vi "imp_test_v7_9215.vi"() -> ()   [LabVIEW 2014]
uses:
  <vilib>/eio/EIONode/EIONode.xnode
  <vilib>/rvi/eio/common/nirviEmuTemplateMethod_errors.vi
  <vilib>/rvi/Analysis/measure/butterworth/XNode/niFpgaButterworthFilter.xnode
  <vilib>/rvi/DataTransferAndStorage/Container/XNode/niFpgaContainer.xnode
  <vilib>/rvi/FXPMathLib/FxpMul/XNode/nifxpmath_Multiplier.xnode
  <vilib>/rvi/FXPMathLib/sim/FxpSim.dll
  <vilib>/rvi/FXPMathLib/FxpSinAndCos/XNode/nifxpmath_SinAndCos.xnode
  <vilib>/rvi/FXPMathLib/FxpSinAndCos/simVIs/DllFxpSinAndCosTemp_sub.vi
  <vilib>/rvi/FXPMathLib/FxpSinAndCos/subVIs/nifxpmath_SinAndCos_SimConfig.ctl
  <vilib>/rvi/FXPMathLib/FxpSub/XNode/nifxpmath_Sub.xnode
  <vilib>/rvi/FXPMathLib/FxpAdd/XNode/nifxpmath_Add.xnode
  <vilib>/rvi/interface/RandomDataEmulation/nirviRandomDataFpgaMultiElementTemplate.vi
panel:
  out "Strain_y (Avg2 w. f)":fxp<+/-,34,7>
  in  "Strain_y Avg2 coeff.":i32[](array[numeric])=[946630756, 63555534]
  out "Strain_y (Avg4 w. f)":fxp<+/-,35,7>
  in  "Strain_y Avg4 coeff.":i32[](array[numeric])=[946630756, 63555534]
  out "Strain_y (Avg2)":fxp<+/-,30,3>
  out "Strain_y (Avg4)":fxp<+/-,31,3>
  in  "Belt_op":fxp<+/-,7,7>
  in  "Belt_mp":fxp<+/-,6,6>
  in  "Belt_oy":fxp<+/-,7,7>
  in  "Belt_my":fxp<+/-,6,6>
  out "Fp_dc":fxp<+/-,32,10>
  out "Fy_dc":fxp<+/-,32,10>
  in  "Zero_y":bool
  in  "Zero_p":bool
  in  "mt0_omega_p":u32
  in  "Encoder reset":bool
  out "fpt_d":fxp<+/-,36,18>
  out "Dp_error_dd":fxp<+/-,36,16>
  out "Dp_error_d":fxp<+/-,33,8>
  in  "Dp_dd coeff.":i32[](array[numeric])=[946630756, 63555534]
  out "Dp_dd":fxp<+/-,36,25>
  out "dFp_PID":fxp<+/-,36,18>
  in  "dFp_PID coeff.":i32[](array[numeric])=[946630756, 63555534]
  out "fpt_i":fxp<+/-,34,18>
  in  "Bv_p":fxp<+/-,22,8>
  in  "Kv_p":fxp<+/-,22,8>
  out "Dp_error":fxp<+/-,22,7>
  out "Dpr_sin":fxp<+/-,22,7>
  in  "Sin offset_p":fxp<+/-,22,7>
  in  "Sin magnitude_p":fxp<+/-,21,6>
  out "Dpr_sin_dd":fxp<+/-,35,20>
  out "Dpr_sin_d":fxp<+/-,33,15>
  out "Sin omega_p":fxp<+/-,34,9>
  in  "Sin wave freq._p (Hz)":fxp<+/-,32,6>
  in  "Dpr_step":fxp<+/-,22,7>
  out "Dpr_for":fxp<+/-,22,7>
  in  "Command_p":i16(ring) items=["Step", "Sine"]
  in  "Ki_p":fxp<+/-,36,9>
  out "Fp_PID":fxp<+/-,36,16>
  in  "fp_tolorance":fxp<+,22,6>
  out "fp_tilde":fxp<+/-,33,10>
  in  "Kd_p":fxp<+/-,36,9>
  in  "Kp_p":fxp<+/-,36,9>
  out "Fr_p":fxp<+/-,32,10>
  in  "S/F coeff_p":fxp<+/-,25,-10>
  in  "S/F coeff_y":fxp<+/-,25,-10>
  out "va_p":fxp<+/-,36,7>
  out "vb_p":fxp<+/-,37,8>
  out "vq_p_F":fxp<+/-,20,5> format="%.57g"
  out "vd_p_F":fxp<+/-,20,5>
  in  "dFp_add":bool
  in  "Stop motor_p":bool
  out "Force_p":fxp<+/-,32,10>
  in  "Strain selection_p":i16(ring) items=["Raw", "Avg.", "Avg. w. filter"]
  out "Strain_p (Avg w. f)":fxp<+/-,36,8>
  in  "Strain_p mean coeff.":i32[](array[numeric])=[946630756, 63555534]
  out "Strain_p (Avg)":fxp<+/-,36,4>
  out "Raw Strain_p":fxp<+/-,36,4>
  out "Mod6/AI3":fxp<+/-,36,4>
  in  "Strain gage reset_p":bool
  out "Dp_d (mm/s)":fxp<+/-,36,11>
  out "omega_p (rad/s)":fxp<+/-,20,9>
  out "mt_omega_p":u32
  out "rad_p(NrTheta)":fxp<+/-,33,20>
  out "D_p(mm)":fxp<+/-,32,7>
  out "Encoder Position_p":i32
  in  "Encoder reset_p":bool
  out "Strain_y (Avg8 w. f)":fxp<+/-,36,8>
  in  "Strain_y Avg8 coeff.":i32[](array[numeric])=[-898916953, 1957103773, 3888751]
  out "Dyr_for":fxp<+/-,22,7>
  in  "Command_y":i16(ring) items=["Step", "Sine"]
  out "Strain_y (Avg8)":fxp<+/-,36,4>
  in  "Strain selection_y":i16(ring) items=["Raw", "Avg.", "Avg. w. filter"]
  out "vb_y":fxp<+/-,38,8>
  out "va_y":fxp<+/-,38,8>
  out "fyt_d":fxp<+/-,36,18>
  out "Fr_y":fxp<+/-,32,10>
  in  "Bv_y":fxp<+/-,22,8>
  out "Dy_error_dd":fxp<+/-,36,16>
  out "Dy_error_d":fxp<+/-,33,8>
  in  "Kv_y":fxp<+/-,22,8>
  out "Dy_error":fxp<+/-,22,7>
  out "Dyr_sin_dd":fxp<+/-,35,20>
  out "Dyr_sin_d":fxp<+/-,33,15>
  out "Sin omega_y":fxp<+/-,34,9>
  out "Dyr_sin":fxp<+/-,22,7>
  in  "Sin offset_y":fxp<+/-,22,7>
  in  "Sin magnitude_y":fxp<+/-,21,6>
  out "Time now(s)":fxp<+,52,14>
  in  "Sin wave freq._y (Hz)":fxp<+/-,32,6>
  in  "Dyr_step":fxp<+/-,22,7>
  in  "Drive mode":i16(ring) items=["Backward", "Forward"]
  out "Dy_dd":fxp<+/-,36,25>
  in  "Dy_dd coeff.":i32[](array[numeric])=[946630756, 63555534]
  out "dFy_PID":fxp<+/-,36,18>
  in  "dFy_PID coeff.":i32[](array[numeric])=[946630756, 63555534]
  out "fyt_i":fxp<+/-,36,16>
  out "Fy_PID":fxp<+/-,36,16>
  in  "fy_tolorance":fxp<+,22,6>
  in  "Ki_y":fxp<+/-,36,9>
  in  "Kd_y":fxp<+/-,36,9>
  out "fy_tilde":fxp<+/-,32,10>
  in  "Kp_y":fxp<+/-,36,9>
  out "vq_y_F":fxp<+/-,20,5> format="%.57g"
  out "vd_y_F":fxp<+/-,20,5>
  in  "dFy_add":bool
  in  "Stop motor_y":bool
  out "Dy_d (mm/s)":fxp<+/-,36,11>
  out "omega_y (rad/s)":fxp<+/-,20,9>
  in  "mt0_omega_y":u32
  out "mt_omega_y":u32
  out "rad_y(NrTheta)":fxp<+/-,33,20>
  out "D_y(mm)":fxp<+/-,32,7>
  out "Encoder Position_y":i32
  in  "Encoder reset_y":bool
  in  "Ini coe.":bool
  out "Loop rate (kHz)":fxp<+/-,36,7>
  out "Force_y":fxp<+/-,32,10>
  out "Raw Strain_y":fxp<+/-,36,4>
  in  "Strain gage reset_y":bool
  out "Mod6/AI2":fxp<+/-,36,4>
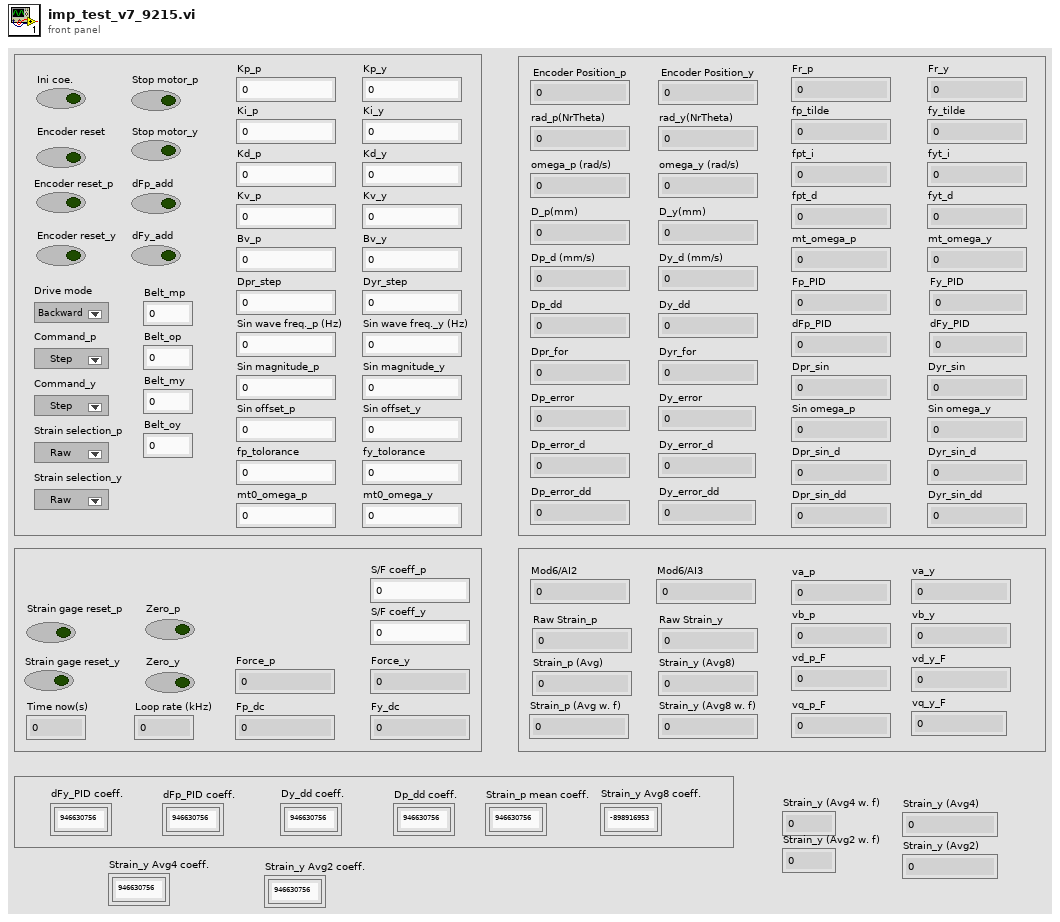
[diagram p1: front panel]
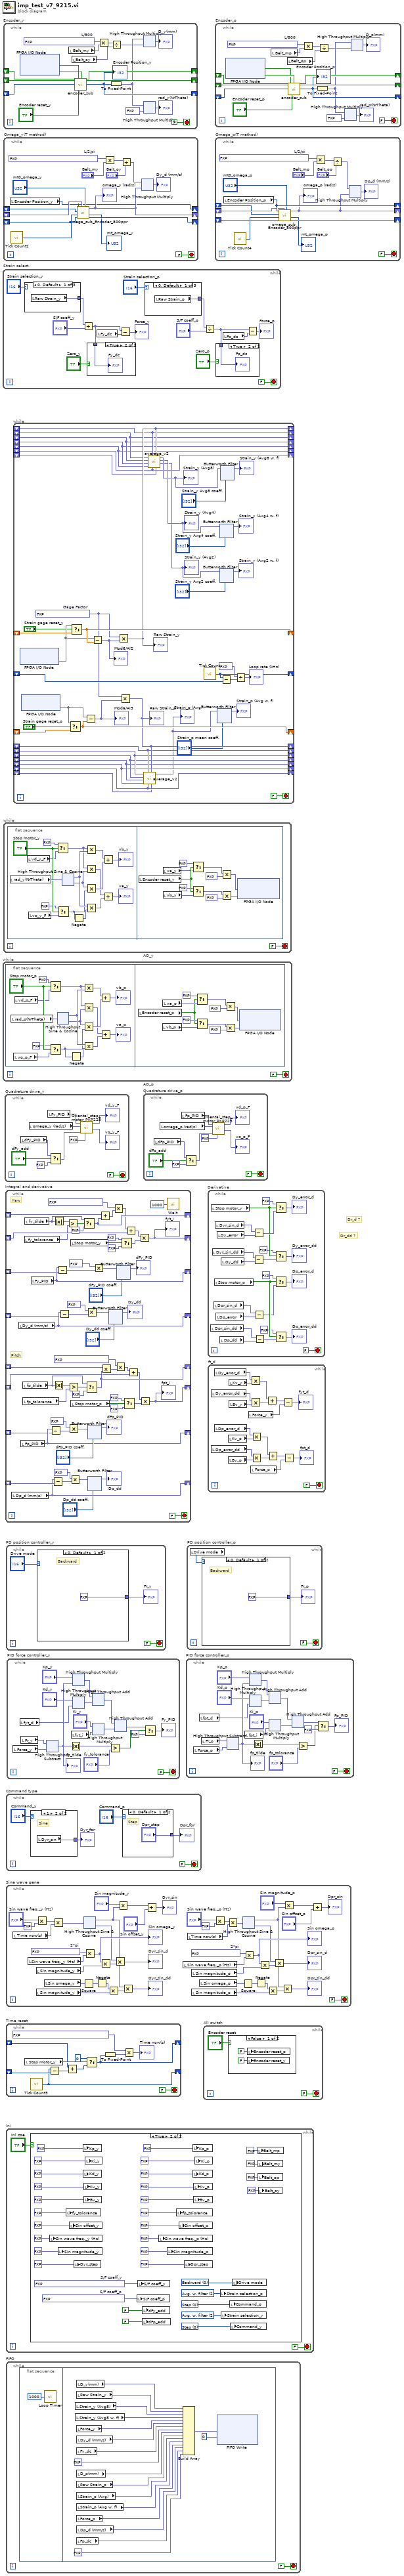
[diagram p0: block diagram]
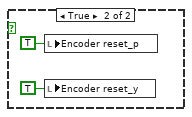
[diagram p2: hidden frame]
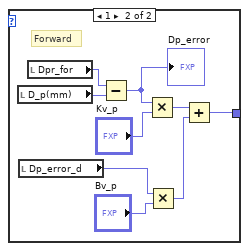
[diagram p3: hidden frame]
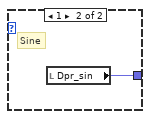
[diagram p4: hidden frame]
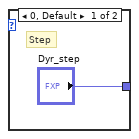
[diagram p5: hidden frame]
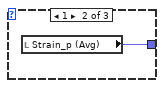
[diagram p8: hidden frame]
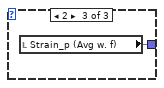
[diagram p9: hidden frame]
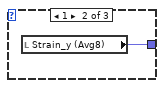
[diagram p10: hidden frame]
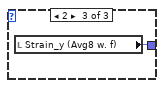
[diagram p11: hidden frame]
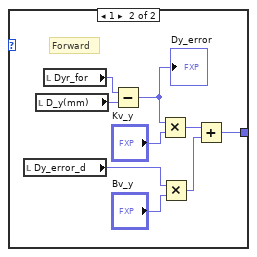
[diagram p12: hidden frame]
diagram:
  # "Dr_dd ?"
  # "Dr_d ?"
  n1 = while "Strain select." {
    stop <- FALSE stop-if-true
    n2 = case shown="0, Default" "Strain selection_y" {
      tunnel: [w21 w22 w23] -> w14
      frame 0, Default {
        n3 = local read "Raw Strain_y"() -> (w21:fxp<+/-,36,4>)
      }
      frame 1 {
        n4 = local read "Strain_y (Avg8)"() -> (w22:fxp<+/-,36,4>)
      }
      frame 2 {
        n5 = local read "Strain_y (Avg8 w. f)"() -> (w23:fxp<+/-,36,8>)
      }
    }
    n6 = Divide(x=w14, y="S/F coeff_y") -> (x/y=w7:fxp<+/-,32,10>)
    n7 = case shown="True" "Zero_y" {
      tunnel: w7 -> [_ w17]
      frame False {
      }
      frame True {
        "Fy_dc" <- w17
      }
    }
    n8 = local read "Fy_dc"() -> (w8:fxp<+/-,32,10>)
    n9 = Subtract(x=w7, y=w8) -> (x-y=→"Force_y":fxp<+/-,33,11>)
    n10 = case shown="0, Default" "Strain selection_p" {
      tunnel: [w18 w19 w20] -> w12
      frame 0, Default {
        n11 = local read "Raw Strain_p"() -> (w18:fxp<+/-,36,4>)
      }
      frame 1 {
        n12 = local read "Strain_p (Avg)"() -> (w19:fxp<+/-,36,4>)
      }
      frame 2 {
        n13 = local read "Strain_p (Avg w. f)"() -> (w20:fxp<+/-,36,8>)
      }
    }
    n14 = Divide(x=w12, y="S/F coeff_p") -> (x/y=w4:fxp<+/-,32,10>)
    n15 = case shown="True" "Zero_p" {
      tunnel: w4 -> [_ w16]
      frame False {
      }
      frame True {
        "Fp_dc" <- w16
      }
    }
    n16 = local read "Fp_dc"() -> (w2:fxp<+/-,32,10>)
    n17 = Subtract(x=w4, y=w2) -> (x-y=→"Force_p":fxp<+/-,33,11>)
  }
  n18 = while "AO_p" {
    stop <- FALSE stop-if-true
    n19 = flat-sequence {
      frame #0 {
        n20 = local read "rad_p(NrTheta)"() -> (w36:fxp<+/-,33,20>)
        n21 = local read "vq_p_F"() -> (w37:fxp<+/-,20,5>)
        n22 = local read "vd_p_F"() -> (w39:fxp<+/-,20,5>)
        n23 = Select(t=fxp<+/-,20,5> 0.0, s="Stop motor_p", f=w39) -> (s? t:f=w28:fxp<+/-,20,5>)
        n24 = Select(t=fxp<+,1,1> 0.0, s="Stop motor_p", f=w37) -> (s? t:f=w27:fxp<+/-,20,5>)
        n25 = xnode "High Throughput Sine & Cosine"("x (pi)"=w36) -> ("sin(x)"=w30:fxp<+/-,16,2>, "cos(x)"=w29:fxp<+/-,16,2>)
        n26 = Negate(x=w27) -> (-x=w35:fxp<+/-,21,6>)
        n27 = Multiply(x=w28, y=w30) -> (x*y=w34:fxp<+/-,36,7>)
        n28 = Multiply(x=w28, y=w29) -> (x*y=w32:fxp<+/-,36,7>)
        n29 = Multiply(x=w29, y=w27) -> (x*y=w33:fxp<+/-,36,7>)
        n30 = Multiply(x=w30, y=w35) -> (x*y=w31:fxp<+/-,35,6>)
        n31 = Add(x=w34, y=w33) -> (x+y=→"vb_p":fxp<+/-,37,8>)
        n32 = Add(x=w32, y=w31) -> (x+y=→"va_p":fxp<+/-,36,7>)
      }
      frame #1 {
        n33 = local read "Encoder reset_p"() -> (w72:bool)
        n34 = local read "vb_p"() -> (w73:fxp<+/-,37,8>)
        n35 = local read "va_p"() -> (w74:fxp<+/-,36,7>)
        n36 = Select(t=fxp<+,2,2> 3.0, s=w72, f=w74) -> (s? t:f=w80:fxp<+/-,36,7>)
        n37 = Select(t=fxp<+,1,1> 0.0, s=w72, f=w73) -> (s? t:f=w79:fxp<+/-,37,8>)
        n38 = Multiply(x=w80, y=fxp<+/-,1,0> -0.5) -> (x*y=w75:fxp<+/-,36,6>)
        n39 = Multiply(x=w79, y=fxp<+/-,1,0> -0.5) -> (x*y=w76:fxp<+/-,36,6>)
        n40 = xnode "FPGA I/O Node"("Mod8/AO0"=w75, "Mod8/AO1"=w76) -> ()  [unwired: 2 in, 2 out]
      }
    }
  }
  n41 = while "Encoder_y" {
    shift-right: [w98] -> _
    shift-left: _ -> [w99]
    shift-right: [w100] -> _
    shift-left: _ -> [w101]
    shift-right: [w93] -> _
    shift-left: _ -> [w97]
    stop <- FALSE stop-if-true
    w87 = fxp<+/-,20,-5> 0.002499997615814209  # L/800
    n42 = xnode "FPGA I/O Node"() -> ("Mod4/DI3"=w96:bool, "Mod4/DI4"=w95:bool)  [unwired: 2 in, 2 out]
    n43 = local read "Belt_my"() -> (w86:fxp<+/-,6,6>)
    n44 = local read "Belt_oy"() -> (w84:fxp<+/-,7,7>)
    n45 = call "encoder_sub.vi"("A_pre"=w99, "B_pre"=w101, "Encoder Position_pre"=w97, "A input"=w96, "Encoder Position Reset"="Encoder reset_y", "B input"=w95) -> ("A"=w98:bool, "B"=w100:bool, "Encoder Position (Counts)"=w93:i32)  [unwired: 19 in]
    "Encoder Position_y" <- w93
    n46 = Multiply(x=w87, y=w86) -> (x*y=w85:fxp<+/-,26,1>)
    n47 = To Fixed-Point(number=w93) -> (fixed-point=w92:fxp<+/-,32,32>)  [unwired: 1 in]
    n48 = Divide(x=w85, y=w84) -> (x/y=w83:fxp<+/-,33,1>)
    n49 = xnode ("High Throughput Multiply")("x"=w92, "y"=w83) -> ("x*y"=→"D_y(mm)":fxp<+/-,64,33>)
    n50 = xnode ("High Throughput Multiply")("x"=w92, "y"=fxp<+/-,16,1> 0.125) -> ("x*y"=→"rad_y(NrTheta)":fxp<+/-,48,33>)
  }
  n51 = while "AO_y" {
    stop <- FALSE stop-if-true
    n52 = flat-sequence {
      frame #0 {
        n53 = local read "rad_y(NrTheta)"() -> (w119:fxp<+/-,33,20>)
        n54 = local read "vd_y_F"() -> (w117:fxp<+/-,20,5>)
        n55 = local read "vq_y_F"() -> (w116:fxp<+/-,20,5>)
        n56 = Select(t=fxp<+/-,20,5> 0.0, s="Stop motor_y", f=w117) -> (s? t:f=w111:fxp<+/-,20,5>)
        n57 = Select(t=fxp<+/-,20,5> 0.0, s="Stop motor_y", f=w116) -> (s? t:f=w110:fxp<+/-,20,5>)
        n58 = xnode "High Throughput Sine & Cosine"("x (pi)"=w119) -> ("sin(x)"=w113:fxp<+/-,17,2>, "cos(x)"=w112:fxp<+/-,17,2>)
        n59 = Negate(x=w110) -> (-x=w109:fxp<+/-,21,6>)
        n60 = Multiply(x=w111, y=w113) -> (x*y=w108:fxp<+/-,37,7>)
        n61 = Multiply(x=w111, y=w112) -> (x*y=w106:fxp<+/-,37,7>)
        n62 = Multiply(x=w112, y=w110) -> (x*y=w107:fxp<+/-,37,7>)
        n63 = Multiply(x=w113, y=w109) -> (x*y=w105:fxp<+/-,36,6>)
        n64 = Add(x=w108, y=w107) -> (x+y=→"vb_y":fxp<+/-,38,8>)
        n65 = Add(x=w106, y=w105) -> (x+y=→"va_y":fxp<+/-,37,7>)
      }
      frame #1 {
        n66 = local read "Encoder reset_y"() -> (w152:bool)
        n67 = local read "va_y"() -> (w151:fxp<+/-,38,8>)
        n68 = local read "vb_y"() -> (w150:fxp<+/-,38,8>)
        n69 = Select(t=fxp<+,2,2> 3.0, s=w152, f=w151) -> (s? t:f=w156:fxp<+/-,38,8>)
        n70 = Select(t=fxp<+,1,1> 0.0, s=w152, f=w150) -> (s? t:f=w155:fxp<+/-,38,8>)
        n71 = Multiply(x=w156, y=fxp<+/-,1,0> -0.5) -> (x*y=w159:fxp<+/-,39,8>)
        n72 = Multiply(x=w155, y=fxp<+/-,1,0> -0.5) -> (x*y=w160:fxp<+/-,37,6>)
        n73 = xnode "FPGA I/O Node"("Mod8/AO2"=w159, "Mod8/AO3"=w160) -> ()  [unwired: 2 in, 2 out]
      }
    }
  }
  n74 = while "Omega_y(T method)" {
    shift-right: [w167] -> _
    shift-left: _ -> [w168]
    shift-right: [w170] -> _
    shift-left: _ -> [w172]
    shift-right: [w174] -> _
    shift-left: _ -> [w175]
    stop <- FALSE stop-if-true
    w165 = fxp<+/-,32,0> 0.3183098859153688  # L/2/pi
    n75 = local read "Encoder Position_y"() -> (w167:i32)
    n76 = call "Tick Count2"() -> ("Tick Count(Ticks)"=w176:u32)
    n77 = call "omega_sub_Encoder_800ppr.vi"("mt0"="mt0_omega_y", "omega_pre"=w172, "ticks_m_pre"=w175, "ticks"=w176, "count_pre"=w168, "count"=w167) -> ("ticks_m"=w174:u32, "mt"=→"mt_omega_y":u32, "omega"=w170:fxp<+/-,20,9>)  [unwired: 3 in]
    "omega_y (rad/s)" <- w170
    n78 = Multiply(x=w165, y="Belt_my") -> (x*y=w163:fxp<+/-,38,6>)
    n79 = Divide(x=w163, y="Belt_oy") -> (x/y=w161:fxp<+/-,20,1>)
    n80 = xnode ("High Throughput Multiply")("x"=w161, "y"=w170) -> ("x*y"=→"Dy_d (mm/s)":fxp<+/-,40,10>)
  }
  n81 = while "Quadrature drive_y" {
    stop <- FALSE stop-if-true
    n82 = local read "dFy_PID"() -> (w178:fxp<+/-,36,18>)
    n83 = local read "omega_y (rad/s)"() -> (w186:fxp<+/-,20,9>)
    n84 = local read "Fy_PID"() -> (w179:fxp<+/-,36,16>)
    n85 = Select(t=w178, s="dFy_add", f=fxp<+,1,1> 0.0) -> (s? t:f=w182:fxp<+/-,36,18>)
    n86 = call "Oriental_step_motor_PKP225.vi"("F_Threshold"=fxp<+,12,12> 10.0, "dFmr"=w182, "omega"=w186, "Fmr"=w179) -> ("vq_F"=→"vq_y_F":fxp<+/-,20,5>, "vd_F"=→"vd_y_F":fxp<+/-,20,5>)  [unwired: 6 in]
  }
  n87 = while "Integral and derivative" {
    shift-right: [w242] -> _
    shift-left: _ -> [w241]
    shift-right: [w234] -> _
    shift-left: _ -> [w233]
    shift-right: [w244] -> _
    shift-left: _ -> [w245]
    shift-right: [w224] -> _
    shift-left: _ -> [w223]
    shift-right: [w210] -> _
    shift-left: _ -> [w213]
    shift-right: [w203] -> _
    shift-left: _ -> [w202]
    shift-right: [w197] -> _
    shift-left: _ -> [w196]
    shift-right: [w192] -> _
    shift-left: _ -> [w193]
    stop <- FALSE stop-if-true
    # "Pitch"
    # "Yaw"
    n88 = local read "Dp_d (mm/s)"() -> (w192:fxp<+/-,36,11>)
    n89 = local read "Dy_d (mm/s)"() -> (w224:fxp<+/-,36,11>)
    n90 = local read "Fp_PID"() -> (w197:fxp<+/-,36,16>)
    n91 = local read "fp_tilde"() -> (w214:fxp<+/-,33,10>)
    n92 = local read "fp_tolorance"() -> (w217:fxp<+,22,6>)
    n93 = local read "fy_tolorance"() -> (w220:fxp<+,22,6>)
    n94 = local read "fy_tilde"() -> (w246:fxp<+/-,32,10>)
    n95 = local read "Fy_PID"() -> (w244:fxp<+/-,36,16>)
    n96 = Subtract(x=w197, y=w196) -> (x-y=w201:fxp<+/-,37,17>)
    n97 = Subtract(x=w192, y=w193) -> (x-y=w194:fxp<+/-,37,12>)
    n98 = Absolute Value(x=w214) -> (abs(x)=w218:fxp<+,33,10>)
    n99 = Absolute Value(x=w246) -> (abs(x)=w248:fxp<+,32,10>)
    n100 = Subtract(x=w244, y=w245) -> (x-y=w232:fxp<+/-,37,17>)
    n101 = Subtract(x=w224, y=w223) -> (x-y=w226:fxp<+/-,36,11>)
    n102 = Greater?(x=w248, y=w220) -> (0:w249:bool)
    n103 = Greater?(x=w218, y=w217) -> (0:w216:bool)
    n104 = Multiply(x=fxp<+,7,10> 1000.0, y=w201) -> (x*y=w199:fxp<+/-,32,18>)
    n105 = Multiply(x=fxp<+,7,10> 1000.0, y=w194) -> (x*y=w190:fxp<+/-,36,21>)
    n106 = local read "Stop motor_y"() -> (w235:bool)
    n107 = local read "Stop motor_p"() -> (w205:bool)
    n108 = Select(t=w246, s=w249, f=fxp<+/-,33,11> 0.0) -> (s? t:f=w242:fxp<+/-,33,11>)
    n109 = Select(t=w214, s=w216, f=fxp<+,1,1> 0.0) -> (s? t:f=w210:fxp<+/-,33,10>)
    n110 = Multiply(x=fxp<+,7,10> 1000.0, y=w226) -> (x*y=w225:fxp<+/-,36,21>)
    n111 = xnode "Butterworth Filter"("input data"=w199, "scaled coefficients"="dFp_PID coeff.") -> ("output data"=→"dFp_PID":fxp<+/-,36,22>)  [unwired: 1 in]
    n112 = xnode "Butterworth Filter"("input data"=w190, "scaled coefficients"="Dp_dd coeff.") -> ("output data"=→"Dp_dd":fxp<+/-,36,25>)  [unwired: 1 in]
    n113 = Multiply(x=fxp<+,7,10> 1000.0, y=w232) -> (x*y=w229:fxp<+/-,32,18>)
    n114 = Add(x=w241, y=w242) -> (x+y=w247:fxp<+/-,34,12>)
    n115 = Multiply(x=w213, y=w210) -> (x*y=w212:fxp<+/-,34,12>)
    n116 = xnode "Butterworth Filter"("input data"=w225, "scaled coefficients"="Dy_dd coeff.") -> ("output data"=→"Dy_dd":fxp<+/-,36,25>)  [unwired: 1 in]
    n117 = Multiply(x=fxp<+/-,30,12> 0.000499725341796875, y=w247) -> (x*y=w240:fxp<+/-,34,10>)
    n118 = Multiply(x=fxp<+/-,30,12> 0.000499725341796875, y=w212) -> (x*y=w209:fxp<+/-,34,10>)
    n119 = xnode "Butterworth Filter"("input data"=w229, "scaled coefficients"="dFy_PID coeff.") -> ("output data"=→"dFy_PID":fxp<+/-,36,22>)  [unwired: 1 in]
    n120 = Select(t=fxp<+,1,1> 0.0, s=w235, f=fxp<+,1,1> 1.0) -> (s? t:f=w238:fxp<+,1,1>)
    n121 = Select(t=fxp<+,1,1> 0.0, s=w205, f=fxp<+,1,1> 1.0) -> (s? t:f=w207:fxp<+,1,1>)
    n122 = Add(x=w240, y=w233) -> (x+y=w239:fxp<+/-,36,16>)
    n123 = Add(x=w209, y=w202) -> (x+y=w208:fxp<+/-,36,16>)
    n124 = Multiply(x=w239, y=w238) -> (x*y=w234:fxp<+/-,34,18>)
    "fyt_i" <- w234
    n125 = Multiply(x=w208, y=w207) -> (x*y=w203:fxp<+/-,34,18>)
    "fpt_i" <- w203
    n126 = call "Wait"("Count(uSec)"=u32 1000) -> ()  [unwired: 1 out]
  }
  n127 = while "PD position controller_y" {
    stop <- FALSE stop-if-true
    n128 = case shown="0, Default" "Drive mode" {
      tunnel: [fxp<+/-,62,19> 0.0 w288] -> w284
      frame 0, Default {
        # "Backward"
      }
      frame 1 {
        # "Forward"
        n129 = local read "Dy_error_d"() -> (w290:fxp<+/-,33,8>)
        n130 = local read "D_y(mm)"() -> (w295:fxp<+/-,32,7>)
        n131 = local read "Dyr_for"() -> (w287:fxp<+/-,22,7>)
        n132 = Subtract(x=w287, y=w295) -> (x-y=w294:fxp<+/-,33,8>)
        "Dy_error" <- w294
        n133 = Multiply(x=w294, y="Kv_y") -> (x*y=w292:fxp<+/-,54,15>)
        n134 = Multiply(x=w290, y="Bv_y") -> (x*y=w289:fxp<+/-,55,16>)
        n135 = Add(x=w292, y=w289) -> (x+y=w288:fxp<+/-,55,16>)
      }
    }
    "Fr_y" <- w284
  }
  n136 = while "Command type" {
    stop <- FALSE stop-if-true
    n137 = case shown="1" "Command_y" {
      tunnel: ["Dyr_step" w304] -> w299
      frame 0, Default {
        # "Step"
      }
      frame 1 {
        # "Sine"
        n138 = local read "Dyr_sin"() -> (w304:fxp<+/-,22,7>)
      }
    }
    "Dyr_for" <- w299
    n139 = case shown="0, Default" "Command_p" {
      tunnel: ["Dpr_step" w302] -> w297
      frame 0, Default {
        # "Step"
      }
      frame 1 {
        # "Sine"
        n140 = local read "Dpr_sin"() -> (w302:fxp<+/-,22,7>)
      }
    }
    "Dpr_for" <- w297
  }
  n141 = while "Sine wave gene" {
    stop <- FALSE stop-if-true
    w310 = fxp<+,20,3> 6.2831878662109375  # 2*pi
    w342 = fxp<+,20,3> 6.2831878662109375  # 2*pi
    n142 = local read "Time now(s)"() -> (w348:fxp<+,52,14>)
    n143 = local read "Sin wave freq._y (Hz)"() -> (w341:fxp<+/-,32,6>)
    n144 = Multiply(x="Sin wave freq._y (Hz)", y=fxp<+/-,10,3> 2.0) -> (x*y=w349:fxp<+/-,41,9>)
    n145 = local read "Sin magnitude_y"() -> (w339:fxp<+/-,21,6>)
    n146 = local read "Sin magnitude_y"() -> (w332:fxp<+/-,21,6>)
    n147 = local read "Sin omega_y"() -> (w335:fxp<+/-,34,9>)
    n148 = Multiply(x=w349, y=w348) -> (x*y=w347:fxp<+/-,41,19>)
    n149 = Square(x=w335) -> (x^2=w334:fxp<+,34,18>)
    n150 = xnode "High Throughput Sine & Cosine"("x (pi)"=w347) -> ("sin(x)"=w329:fxp<+/-,16,2>, "cos(x)"=w337:fxp<+/-,16,2>)
    n151 = Multiply(x=w342, y=w341) -> (x*y=w340:fxp<+/-,34,9>)
    "Sin omega_y" <- w340
    n152 = Negate(x=w334) -> (-x=w333:fxp<+/-,35,19>)
    n153 = Multiply(x=w340, y=w339) -> (x*y=w338:fxp<+/-,33,15>)
    n154 = Multiply(x=w333, y=w332) -> (x*y=w331:fxp<+/-,34,20>)
    n155 = Multiply(x=w337, y=w338) -> (x*y=→"Dyr_sin_d":fxp<+/-,33,15>)
    n156 = Multiply(x="Sin magnitude_y", y=w329) -> (x*y=w345:fxp<+/-,37,8>)
    n157 = Multiply(x=w329, y=w331) -> (x*y=→"Dyr_sin_dd":fxp<+/-,35,20>)
    n158 = Add(x=w345, y="Sin offset_y") -> (x+y=→"Dyr_sin":fxp<+/-,37,8>)
    n159 = local read "Sin wave freq._p (Hz)"() -> (w306:fxp<+/-,32,6>)
    n160 = local read "Time now(s)"() -> (w324:fxp<+,52,14>)
    n161 = local read "Sin magnitude_p"() -> (w307:fxp<+/-,21,6>)
    n162 = local read "Sin magnitude_p"() -> (w309:fxp<+/-,21,6>)
    n163 = local read "Sin omega_p"() -> (w308:fxp<+/-,34,9>)
    n164 = Multiply(x="Sin wave freq._p (Hz)", y=fxp<+/-,10,3> 2.0) -> (x*y=w328:fxp<+/-,42,9>)
    n165 = Multiply(x=w328, y=w324) -> (x*y=w325:fxp<+/-,41,19>)
    n166 = Square(x=w308) -> (x^2=w320:fxp<+,34,18>)
    n167 = xnode "High Throughput Sine & Cosine"("x (pi)"=w325) -> ("sin(x)"=w311:fxp<+/-,16,2>, "cos(x)"=w316:fxp<+/-,16,2>)
    n168 = Multiply(x=w310, y=w306) -> (x*y=w323:fxp<+/-,34,9>)
    "Sin omega_p" <- w323
    n169 = Negate(x=w320) -> (-x=w319:fxp<+/-,35,19>)
    n170 = Multiply(x=w323, y=w307) -> (x*y=w322:fxp<+/-,33,15>)
    n171 = Multiply(x=w319, y=w309) -> (x*y=w318:fxp<+/-,35,19>)
    n172 = Multiply(x=w316, y=w322) -> (x*y=→"Dpr_sin_d":fxp<+/-,33,15>)
    n173 = Multiply(x=w311, y=w318) -> (x*y=→"Dpr_sin_dd":fxp<+/-,35,20>)
    n174 = Multiply(x="Sin magnitude_p", y=w311) -> (x*y=w314:fxp<+/-,37,8>)
    n175 = Add(x=w314, y="Sin offset_p") -> (x+y=→"Dpr_sin":fxp<+/-,37,8>)
  }
  n176 = while "Time reset" {
    shift-right: [w421] -> _
    shift-left: _ -> [w422]
    shift-right: [w416] -> _
    shift-left: _ -> [w417]
    stop <- FALSE stop-if-true
    n177 = local read "Stop motor_y"() -> (w423:bool)
    n178 = call "Tick Count3"() -> ("Tick Count(uSec)"=w421:u32)
    n179 = Subtract(x=w421, y=w422) -> (x-y=w420:u32)
    n180 = Add(x=w417, y=w420) -> (x+y=w419:u32)
    n181 = Select(t=u32 0, s=w423, f=w419) -> (s? t:f=w416:u32)
    n182 = To Fixed-Point(number=w416) -> (fixed-point=w415:fxp<+,32,32>)  [unwired: 1 in]
    n183 = Multiply(x=fxp<+,20,-18> 1.0000003385357559e-06, y=w415) -> (x*y=→"Time now(s)":fxp<+,52,14>)
  }
  n184 = while "Ini" {
    stop <- FALSE stop-if-true
    n185 = case shown="True" "Ini coe." {
      frame False {
      }
      frame True {
        w441 = i16 0 items=["Step", "Sine"] ("Command_p")
        w442 = i16 2 items=["Raw", "Avg.", "Avg. w. filter"] ("Strain selection_p")
        w443 = i16 0 items=["Step", "Sine"] ("Command_y")
        w444 = i16 2 items=["Raw", "Avg.", "Avg. w. filter"] ("Strain selection_y")
        w446 = fxp<+/-,25,-10> -5.851034075021744e-07  # S/F coeff_p
        w445 = fxp<+/-,25,-10> -1.0477961041033268e-06  # S/F coeff_y
        w452 = i16 0 items=["Backward", "Forward"] ("Drive mode")
        n186 = local write "Sin wave freq._y (Hz)"(fxp<+/-,32,6> 1.0 ("Sin wave freq. (Hz)")) -> ()
        n187 = local write "Sin magnitude_y"(fxp<+/-,22,7> 5.0 ("Sin magnitude")) -> ()
        n188 = local write "fy_tolorance"(fxp<+,22,6> 5.0 ("f_tolorance")) -> ()
        n189 = local write "Sin offset_y"(fxp<+/-,38,9> 0.0 ("Sin offset")) -> ()
        n190 = local write "Dyr_step"(fxp<+/-,22,7> 0.0 ("Dr")) -> ()
        n191 = local write "Kp_y"(fxp<+/-,36,9> 30.0 ("Kp")) -> ()
        n192 = local write "Kd_y"(fxp<+/-,36,9> 0.0 ("Kd")) -> ()
        n193 = local write "Kv_y"(fxp<+/-,22,8> 0.0 ("Kv")) -> ()
        n194 = local write "Bv_y"(fxp<+/-,22,8> 0.0 ("Bv")) -> ()
        n195 = local write "Ki_y"(fxp<+/-,36,9> 0.0 ("Ki")) -> ()
        n196 = local write "S/F coeff_p"(w446) -> ()
        n197 = local write "S/F coeff_y"(w445) -> ()
        n198 = local write "dFy_add"(FALSE ("dF_add")) -> ()
        n199 = local write "dFp_add"(FALSE ("dFp_add")) -> ()
        n200 = local write "Sin wave freq._p (Hz)"(fxp<+/-,32,6> 1.0 ("Sin wave freq._p (Hz)")) -> ()
        n201 = local write "Sin magnitude_p"(fxp<+/-,21,6> 5.0 ("Sin magnitude_p")) -> ()
        n202 = local write "fp_tolorance"(fxp<+,22,6> 5.0 ("fp_tolorance")) -> ()
        n203 = local write "Sin offset_p"(fxp<+/-,22,7> 0.0 ("Sin offset_p")) -> ()
        n204 = local write "Dpr_step"(fxp<+/-,22,7> 0.0 ("Dpr_step")) -> ()
        n205 = local write "Kp_p"(fxp<+/-,36,9> 30.0 ("Kp_p")) -> ()
        n206 = local write "Kd_p"(fxp<+/-,36,9> 0.0 ("Kd_p")) -> ()
        n207 = local write "Kv_p"(fxp<+/-,22,8> 0.0 ("Kv_p")) -> ()
        n208 = local write "Bv_p"(fxp<+/-,22,8> 0.0 ("Bv_p")) -> ()
        n209 = local write "Ki_p"(fxp<+/-,36,9> 0.0 ("Ki_p")) -> ()
        n210 = local write "Strain selection_p"(w442) -> ()
        n211 = local write "Strain selection_y"(w444) -> ()
        n212 = local write "Command_p"(w441) -> ()
        n213 = local write "Command_y"(w443) -> ()
        n214 = local write "Drive mode"(w452) -> ()
        n215 = local write "Belt_mp"(fxp<+/-,6,6> 16.0 ("Belt_mp")) -> ()
        n216 = local write "Belt_my"(fxp<+/-,6,6> 22.0 ("Belt_my")) -> ()
        n217 = local write "Belt_op"(fxp<+/-,7,7> 16.0 ("Belt_op")) -> ()
        n218 = local write "Belt_oy"(fxp<+/-,7,7> 22.0 ("Belt_oy")) -> ()
      }
    }
  }
  n219 = while "FIFO" {
    stop <- FALSE stop-if-true
    n220 = flat-sequence {
      frame #0 {
        n221 = call "Loop Timer"("Count(uSec)"=u32 1000) -> ()  [unwired: 1 out]
      }
      frame #1 {
        n222 = local read "Strain_y (Avg8)"() -> (w476:fxp<+/-,36,4>)
        n223 = local read "Strain_y (Avg8 w. f)"() -> (w475:fxp<+/-,36,8>)
        n224 = local read "D_y(mm)"() -> (w478:fxp<+/-,32,7>)
        n225 = local read "Raw Strain_y"() -> (w477:fxp<+/-,36,4>)
        n226 = local read "Force_y"() -> (w470:fxp<+/-,32,10>)
        n227 = local read "Dy_d (mm/s)"() -> (w471:fxp<+/-,36,11>)
        n228 = local read "Fy_dc"() -> (w472:fxp<+/-,32,10>)
        n229 = local read "D_p(mm)"() -> (w469:fxp<+/-,32,7>)
        n230 = local read "Raw Strain_p"() -> (w468:fxp<+/-,36,4>)
        n231 = local read "Strain_p (Avg)"() -> (w467:fxp<+/-,36,4>)
        n232 = local read "Strain_p (Avg w. f)"() -> (w466:fxp<+/-,36,8>)
        n233 = local read "Force_p"() -> (w465:fxp<+/-,32,10>)
        n234 = local read "Dp_d (mm/s)"() -> (w464:fxp<+/-,36,11>)
        n235 = local read "Fp_dc"() -> (w463:fxp<+/-,32,10>)
        n236 = Build Array(w478, w477, w476, w475, w470, w471, w472, fxp<+/-,40,8> 0.0 ("element"), w469, w468, w467, w466, w465, w464, w463, fxp<+/-,40,8> 0.0 ("element")) -> (w461:fxp<+/-,43,11>[])
        n237 = xnode ("FIFO Write")("Element"=w461, "Timeout"=0) -> ()  [unwired: 1 in, 2 out]
      }
    }
  }
  n238 = while "PID force controller_y" {
    stop <- FALSE stop-if-true
    n239 = local read "Force_y"() -> (w496:fxp<+/-,32,10>)
    n240 = local read "fyt_d"() -> (w480:fxp<+/-,36,18>)
    n241 = local read "Fr_y"() -> (w482:fxp<+/-,32,10>)
    n242 = xnode "High Throughput Subtract"("x"=w482, "y"=w496) -> ("x-y"=w495:fxp<+/-,33,11>)
    "fy_tilde" <- w495
    n243 = Absolute Value(x=w495) -> (abs(x)=w486:fxp<+,33,11>)
    n244 = local read "fyt_i"() -> (w481:fxp<+/-,36,16>)
    n245 = xnode ("High Throughput Multiply")("x"="Kp_y", "y"=w495) -> ("x*y"=w493:fxp<+/-,64,20>)
    n246 = xnode ("High Throughput Multiply")("x"="Kd_y", "y"=w480) -> ("x*y"=w492:fxp<+/-,64,27>)
    n247 = xnode ("High Throughput Add")("x"=w493, "y"=w492) -> ("x+y"=w489:fxp<+/-,64,28>)
    n248 = xnode ("High Throughput Multiply")("x"="Ki_y", "y"=w481) -> ("x*y"=w490:fxp<+/-,64,25>)
    n249 = Greater?(x=w486, y="fy_tolorance") -> (0:w484:bool)
    n250 = xnode ("High Throughput Add")("x"=w489, "y"=w490) -> ("x+y"=w488:fxp<+/-,64,29>)
    n251 = Select(t=w488, s=w484, f=fxp<+/-,51,14> 0.0) -> (s? t:f=→"Fy_PID":fxp<+/-,64,29>)
  }
  n252 = while {
    shift-right: [w541] -> _
    shift-left: _ -> [w542]
    shift-right: [w537] -> _
    shift-left: _ -> [w538]
    shift-right: [w532] -> _
    shift-left: _ -> [w531]
    shift-right: [w531] -> _
    shift-left: _ -> [w530]
    shift-right: [w530] -> _
    shift-left: _ -> [w529]
    shift-right: [w529] -> _
    shift-left: _ -> [w528]
    shift-right: [w528] -> _
    shift-left: _ -> [w527]
    shift-right: [w527] -> _
    shift-left: _ -> [w526]
    shift-right: [w526] -> _
    shift-left: _ -> [w525]
    shift-right: [w519] -> _
    shift-left: _ -> [w520]
    shift-right: [w515] -> _
    shift-left: _ -> [w514]
    shift-right: [w514] -> _
    shift-left: _ -> [w513]
    shift-right: [w513] -> _
    shift-left: _ -> [w512]
    shift-right: [w512] -> _
    shift-left: _ -> [w511]
    shift-right: [w511] -> _
    shift-left: _ -> [w510]
    shift-right: [w510] -> _
    shift-left: _ -> [w509]
    shift-right: [w509] -> _
    shift-left: _ -> [w508]
    stop <- FALSE stop-if-true
    w517 = fxp<+,20,2> 2.115001678466797  # Gage Factor
    n253 = xnode "FPGA I/O Node"() -> ("Mod1/AI1"=w539)  [unwired: 2 in, 2 out]
    n254 = xnode "FPGA I/O Node"() -> ("Mod1/AI2"=w518)  [unwired: 2 in, 2 out]
    n255 = Select(t=w518, s="Strain gage reset_p", f=w520) -> (s? t:f=w519:dbl)
    n256 = Select(t=w539, s="Strain gage reset_y", f=w542) -> (s? t:f=w541:dbl)
    n257 = Subtract(x=w518, y=w519) -> (x-y=w516:fxp<+/-,30,-3>)
    "Mod6/AI3" <- w516
    n258 = Subtract(x=w539, y=w541) -> (x-y=w540:fxp<+/-,30,-3>)
    "Mod6/AI2" <- w540
    n259 = Multiply(x=w517, y=w540) -> (x*y=w532:fxp<+/-,41,6>)
    "Raw Strain_y" <- w532
    n260 = Multiply(x=w517, y=w516) -> (x*y=w515:fxp<+/-,50,-1>)
    "Raw Strain_p" <- w515
    n261 = call "average_v2.vi"("Numeric 8"=w508, "Numeric"=w515, "Numeric 7"=w509, "Numeric 2"=w514, "Numeric 6"=w510, "Numeric 5"=w511, "Numeric 4"=w512, "Numeric 3"=w513) -> ("Mean (8pt)"=w507:fxp<+/-,32,4>)  [unwired: 1 in, 2 out]
    "Strain_p (Avg)" <- w507
    n262 = call "average_v2.vi"("Numeric 8"=w525, "Numeric"=w532, "Numeric 7"=w526, "Numeric 2"=w531, "Numeric 6"=w527, "Numeric 5"=w528, "Numeric 4"=w529, "Numeric 3"=w530) -> ("Mean (2pt)"=w501:fxp<+/-,30,3>, "Mean (4pt)"=w504:fxp<+/-,31,3>, "Mean (8pt)"=w524:fxp<+/-,32,4>)  [unwired: 1 in]
    "Strain_y (Avg8)" <- w524
    "Strain_y (Avg4)" <- w504
    "Strain_y (Avg2)" <- w501
    n263 = call "Tick Count"() -> ("Tick Count(uSec)"=w537:u32)
    n264 = xnode "Butterworth Filter"("input data"=w507, "scaled coefficients"="Strain_p mean coeff.") -> ("output data"=→"Strain_p (Avg w. f)":fxp<+/-,36,8>)  [unwired: 1 in]
    n265 = xnode "Butterworth Filter"("input data"=w504, "scaled coefficients"="Strain_y Avg4 coeff.") -> ("output data"=→"Strain_y (Avg4 w. f)":fxp<+/-,35,7>)  [unwired: 1 in]
    n266 = xnode "Butterworth Filter"("input data"=w501, "scaled coefficients"="Strain_y Avg2 coeff.") -> ("output data"=→"Strain_y (Avg2 w. f)":fxp<+/-,34,7>)  [unwired: 1 in]
    n267 = xnode "Butterworth Filter"("input data"=w524, "scaled coefficients"="Strain_y Avg8 coeff.") -> ("output data"=→"Strain_y (Avg8 w. f)":fxp<+/-,32,4>)  [unwired: 1 in]
    n268 = Subtract(x=w537, y=w538) -> (x-y=w535:fxp<+/-,32,16>)
    n269 = Divide(x=fxp<+,7,10> 1000.0, y=w535) -> (x/y=→"Loop rate (kHz)":fxp<+/-,40,27>)
  }
  n270 = while "Quadrature drive_p" {
    stop <- FALSE stop-if-true
    n271 = local read "dFp_PID"() -> (w576:fxp<+/-,36,18>)
    n272 = local read "omega_p (rad/s)"() -> (w582:fxp<+/-,20,9>)
    n273 = local read "Fp_PID"() -> (w577:fxp<+/-,36,16>)
    n274 = Select(t=w576, s="dFp_add", f=fxp<+,1,1> 0.0) -> (s? t:f=w580:fxp<+/-,36,18>)
    n275 = call "Oriental_step_motor_PKP225.vi"("F_Threshold"=fxp<+,12,12> 10.0, "dFmr"=w580, "omega"=w582, "Fmr"=w577) -> ("vq_F"=→"vq_p_F":fxp<+/-,20,5>, "vd_F"=→"vd_p_F":fxp<+/-,20,5>)  [unwired: 6 in]
  }
  n276 = while "PID force controller_p" {
    stop <- FALSE stop-if-true
    n277 = local read "Force_p"() -> (w597:fxp<+/-,32,10>)
    n278 = local read "fpt_d"() -> (w588:fxp<+/-,36,18>)
    n279 = local read "Fr_p"() -> (w598:fxp<+/-,32,10>)
    n280 = xnode "High Throughput Subtract"("x"=w598, "y"=w597) -> ("x-y"=w589:fxp<+/-,33,11>)
    "fp_tilde" <- w589
    n281 = local read "fpt_i"() -> (w586:fxp<+/-,34,18>)
    n282 = xnode ("High Throughput Multiply")("x"="Kp_p", "y"=w589) -> ("x*y"=w587:fxp<+/-,64,20>)
    n283 = xnode ("High Throughput Multiply")("x"="Kd_p", "y"=w588) -> ("x*y"=w603:fxp<+/-,64,27>)
    n284 = Absolute Value(x=w589) -> (abs(x)=w596:fxp<+,33,11>)
    n285 = xnode ("High Throughput Add")("x"=w587, "y"=w603) -> ("x+y"=w601:fxp<+/-,64,28>)
    n286 = xnode ("High Throughput Multiply")("x"="Ki_p", "y"=w586) -> ("x*y"=w602:fxp<+/-,64,27>)
    n287 = xnode ("High Throughput Add")("x"=w601, "y"=w602) -> ("x+y"=w592:fxp<+/-,64,29>)
    n288 = Greater?(x=w596, y="fp_tolorance") -> (0:w593:bool)
    n289 = Select(t=w592, s=w593, f=fxp<+,1,1> 0.0) -> (s? t:f=→"Fp_PID":fxp<+/-,64,29>)
  }
  n290 = while "PD position controller_p" {
    stop <- FALSE stop-if-true
    n291 = local read "Drive mode"() -> (w606:i16)
    n292 = case shown="0, Default" w606 {
      tunnel: [fxp<+/-,62,19> 0.0 w609] -> w605
      frame 0, Default {
        # "Backward"
      }
      frame 1 {
        # "Forward"
        n293 = local read "D_p(mm)"() -> (w616:fxp<+/-,32,7>)
        n294 = local read "Dp_error_d"() -> (w608:fxp<+/-,33,8>)
        n295 = local read "Dpr_for"() -> (w615:fxp<+/-,22,7>)
        n296 = Subtract(x=w615, y=w616) -> (x-y=w614:fxp<+/-,24,8>)
        "Dp_error" <- w614
        n297 = Multiply(x=w614, y="Kv_p") -> (x*y=w611:fxp<+/-,34,16>)
        n298 = Multiply(x=w608, y="Bv_p") -> (x*y=w610:fxp<+/-,55,16>)
        n299 = Add(x=w611, y=w610) -> (x+y=w609:fxp<+/-,56,17>)
      }
    }
    "Fr_p" <- w605
  }
  n300 = while "All switch" {
    stop <- FALSE stop-if-true
    n301 = case shown="False" "Encoder reset" {
      frame False {
        n302 = local write "Encoder reset_p"(FALSE ("Encoder reset_p")) -> ()
        n303 = local write "Encoder reset_y"(FALSE ("Encoder reset_y")) -> ()
      }
      frame True {
        n304 = local write "Encoder reset_p"(TRUE ("Encoder reset_p")) -> ()
        n305 = local write "Encoder reset_y"(TRUE ("Encoder reset_y")) -> ()
      }
    }
  }
  n306 = while "Derivative" {
    stop <- FALSE stop-if-true
    n307 = local read "Dpr_sin_dd"() -> (w631:fxp<+/-,35,20>)
    n308 = local read "Stop motor_y"() -> (w637:bool)
    n309 = local read "Dyr_sin_dd"() -> (w639:fxp<+/-,35,20>)
    n310 = local read "Dpr_sin_d"() -> (w633:fxp<+/-,33,15>)
    n311 = local read "Stop motor_p"() -> (w629:bool)
    n312 = local read "Dyr_sin_d"() -> (w642:fxp<+/-,33,15>)
    n313 = local read "Dp_error"() -> (w634:fxp<+/-,22,7>)
    n314 = local read "Dy_error"() -> (w643:fxp<+/-,22,7>)
    n315 = local read "Dp_dd"() -> (w632:fxp<+/-,36,25>)
    n316 = local read "Dy_dd"() -> (w640:fxp<+/-,36,25>)
    n317 = Subtract(x=w642, y=w643) -> (x-y=w641:fxp<+/-,34,16>)
    n318 = Subtract(x=w639, y=w640) -> (x-y=w638:fxp<+/-,41,26>)
    n319 = Subtract(x=w633, y=w634) -> (x-y=w626:fxp<+/-,34,16>)
    n320 = Subtract(x=w631, y=w632) -> (x-y=w630:fxp<+/-,41,26>)
    n321 = Select(t=fxp<+,1,1> 0.0, s=w637, f=w641) -> (s? t:f=→"Dy_error_d":fxp<+/-,34,16>)
    n322 = Select(t=fxp<+/-,64,49> 0.0, s=w637, f=w638) -> (s? t:f=→"Dy_error_dd":fxp<+/-,64,49>)
    n323 = Select(t=fxp<+,1,1> 0.0, s=w629, f=w626) -> (s? t:f=→"Dp_error_d":fxp<+/-,34,16>)
    n324 = Select(t=fxp<+/-,41,26> 0.0, s=w629, f=w630) -> (s? t:f=→"Dp_error_dd":fxp<+/-,41,26>)
  }
  n325 = while "ft_d" {
    stop <- FALSE stop-if-true
    n326 = local read "Dy_error_dd"() -> (w661:fxp<+/-,36,16>)
    n327 = local read "Dp_error_dd"() -> (w652:fxp<+/-,36,16>)
    n328 = local read "Dy_error_d"() -> (w663:fxp<+/-,33,8>)
    n329 = local read "Dp_error_d"() -> (w654:fxp<+/-,33,8>)
    n330 = local read "Kv_p"() -> (w655:fxp<+/-,22,8>)
    n331 = local read "Bv_p"() -> (w653:fxp<+/-,22,8>)
    n332 = local read "Kv_y"() -> (w664:fxp<+/-,22,8>)
    n333 = local read "Bv_y"() -> (w662:fxp<+/-,22,8>)
    n334 = local read "Force_y"() -> (w657:fxp<+/-,32,10>)
    n335 = Multiply(x=w663, y=w664) -> (x*y=w659:fxp<+/-,55,16>)
    n336 = Multiply(x=w661, y=w662) -> (x*y=w660:fxp<+/-,58,24>)
    n337 = Multiply(x=w654, y=w655) -> (x*y=w650:fxp<+/-,55,16>)
    n338 = Multiply(x=w652, y=w653) -> (x*y=w651:fxp<+/-,58,24>)
    n339 = local read "Force_p"() -> (w648:fxp<+/-,32,10>)
    n340 = Add(x=w659, y=w660) -> (x+y=w658:fxp<+/-,63,24>)
    n341 = Add(x=w650, y=w651) -> (x+y=w649:fxp<+/-,63,24>)
    n342 = Subtract(x=w658, y=w657) -> (x-y=→"fyt_d":fxp<+/-,63,24>)
    n343 = Subtract(x=w649, y=w648) -> (x-y=→"fpt_d":fxp<+/-,63,24>)
  }
  n344 = while "Encoder_p" {
    shift-right: [w679] -> _
    shift-left: _ -> [w680]
    shift-right: [w681] -> _
    shift-left: _ -> [w682]
    shift-right: [w675] -> _
    shift-left: _ -> [w683]
    stop <- FALSE stop-if-true
    w669 = fxp<+/-,20,-5> 0.002499997615814209  # L/800
    n345 = xnode "FPGA I/O Node"() -> ("Mod4/DI0"=w677:bool, "Mod4/DI1"=w678:bool)  [unwired: 2 in, 2 out]
    n346 = local read "Belt_mp"() -> (w668:fxp<+/-,6,6>)
    n347 = local read "Belt_op"() -> (w666:fxp<+/-,7,7>)
    n348 = call "encoder_sub.vi"("A_pre"=w680, "B_pre"=w682, "Encoder Position_pre"=w683, "A input"=w677, "Encoder Position Reset"="Encoder reset_p", "B input"=w678) -> ("A"=w679:bool, "B"=w681:bool, "Encoder Position (Counts)"=w675:i32)  [unwired: 19 in]
    "Encoder Position_p" <- w675
    n349 = Multiply(x=w669, y=w668) -> (x*y=w667:fxp<+/-,26,1>)
    n350 = To Fixed-Point(number=w675) -> (fixed-point=w674:fxp<+/-,32,32>)  [unwired: 1 in]
    n351 = Divide(x=w667, y=w666) -> (x/y=w665:fxp<+/-,33,1>)
    n352 = xnode ("High Throughput Multiply")("x"=w674, "y"=fxp<+/-,16,1> 0.125) -> ("x*y"=→"rad_p(NrTheta)":fxp<+/-,48,33>)
    n353 = xnode ("High Throughput Multiply")("x"=w674, "y"=w665) -> ("x*y"=→"D_p(mm)":fxp<+/-,64,33>)
  }
  n354 = while "Omega_p(T method)" {
    shift-right: [w699] -> _
    shift-left: _ -> [w697]
    shift-right: [w692] -> _
    shift-left: _ -> [w698]
    shift-right: [w694] -> _
    shift-left: _ -> [w696]
    stop <- FALSE stop-if-true
    w688 = fxp<+/-,32,0> 0.3183098859153688  # L/2/pi
    n355 = local read "Encoder Position_p"() -> (w699:i32)
    n356 = call "Tick Count4"() -> ("Tick Count(Ticks)"=w695:u32)
    n357 = call "omega_sub_Encoder_800ppr.vi"("mt0"="mt0_omega_p", "omega_pre"=w698, "ticks_m_pre"=w696, "ticks"=w695, "count_pre"=w697, "count"=w699) -> ("ticks_m"=w694:u32, "mt"=→"mt_omega_p":u32, "omega"=w692:fxp<+/-,20,9>)  [unwired: 3 in]
    "omega_p (rad/s)" <- w692
    n358 = Multiply(x=w688, y="Belt_mp") -> (x*y=w686:fxp<+/-,38,6>)
    n359 = Divide(x=w686, y="Belt_op") -> (x/y=w684:fxp<+/-,20,1>)
    n360 = xnode ("High Throughput Multiply")("x"=w684, "y"=w692) -> ("x*y"=→"Dp_d (mm/s)":fxp<+/-,40,10>)
  }
